vi "Helium Fridge Cool-Down.vi"() -> ()   [LabVIEW 2014]
uses:
  <vilib>/Analysis/8numeric.llb/1D Numeric Integration.vi
  <vilib>/express/express shared/transition.llb/Dynamic To Waveform Array.vi
  <vilib>/express/express signal manip/GetorSetDDTAttributes/Set DDT Attributes/SetT0.vi
  <vilib>/express/express shared/transition.llb/Waveform Array To Dynamic.vi
  <vilib>/express/express signal manip/GetorSetDDTAttributes/Set DDT Attributes/Set DDT Properties.xnode
  <vilib>/Analysis/NI_AALPro.lvlib
panel:
  out "Numeric Indicator":dbl
  in  "Depth/Div Submit":bool
  out "Depth/Div (kHz)":dbl
  in  "Cent. Frq. Submit":bool
  out "Cent. Freq. (MHz)":dbl
  out "Temp 2":bool
  out "Temperature Strip Chart":dynamicdata(graph)
  in  "TC Points/Measurement":dbl=20.0
  out "NMR":bool
  out "NMR Temp Error":bool
  out "Q Meter Temp":dynamicdata(graph)
  out "Zeroed Array":dbl[](array[numeric])
  out "Fit X values":dbl[](array[numeric])
  in  "Left wing 2":dbl
  in  "Right wing 2":dbl
  in  "Right wing":dbl
  in  "Left wing":dbl
  out "Fit":dbl[](array[numeric])
  in  "Submit":bool
  out "Is Flashing":bool
  in  "Error Beat":bool
  in  "Clear":bool
  in  "Comment":string
  out "Heartbeat":bool
  out "Most Recent Error":string
  out "Baseline Subtracted Integral vs. Time":dbl(graph)
  out "Time of Last Baseline":string
  out "Baseline":dbl[](array[numeric])
  in  "Baseline Subtract":bool
  in  "Get Baseline":bool
  out "Recording":bool
  out "Time of Last Recording":string
  in  "Record \nNMR Sweeps":bool
  in  "Depth/Div\n(MHz)":dbl=10.0
  in  "Central Freq. \n(MHz)":dbl=13.0
  in  "stop (F)":bool caption="Triangle Wave"
  in  "Triangle Wave\nRate (Hz)":dbl=0.3
  out "Time Elapsed \nDuring Sweeps (s)":dbl
  out "Lab Time":string
  out "Most Recent Error (NMR)":string
  out "Last Sweep Start Time":string
  out "Most Recent Error (Temp)":string
  out "Last Measurement Taken":string
  out "VI Start Time":string
  in  "Time Between\nTemp Ponts (s)":dbl=30.0
  out "Temp":bool
  out "NMR":bool
  in  "stop":bool
  out "Input Triangle Wave":dynamicdata(graph)
  out "Modulator":dynamicdata(graph)
  out "NMR":cluster{"Y":dbl[], "Y":dbl[]}[](graph)
  in  "# of Sweeps":dbl=1.0
  out "Resistance Strip Chart":dynamicdata(graph)
  in  "Heartbeat":bool
  in  "Temp Strip Chart":bool
  out "Errors":bool
  in  "Silence Flashing":bool
  # "Initialization and Logic Controls -- DO NOT TOUCH!!"
  # "Caitlyn's Work"
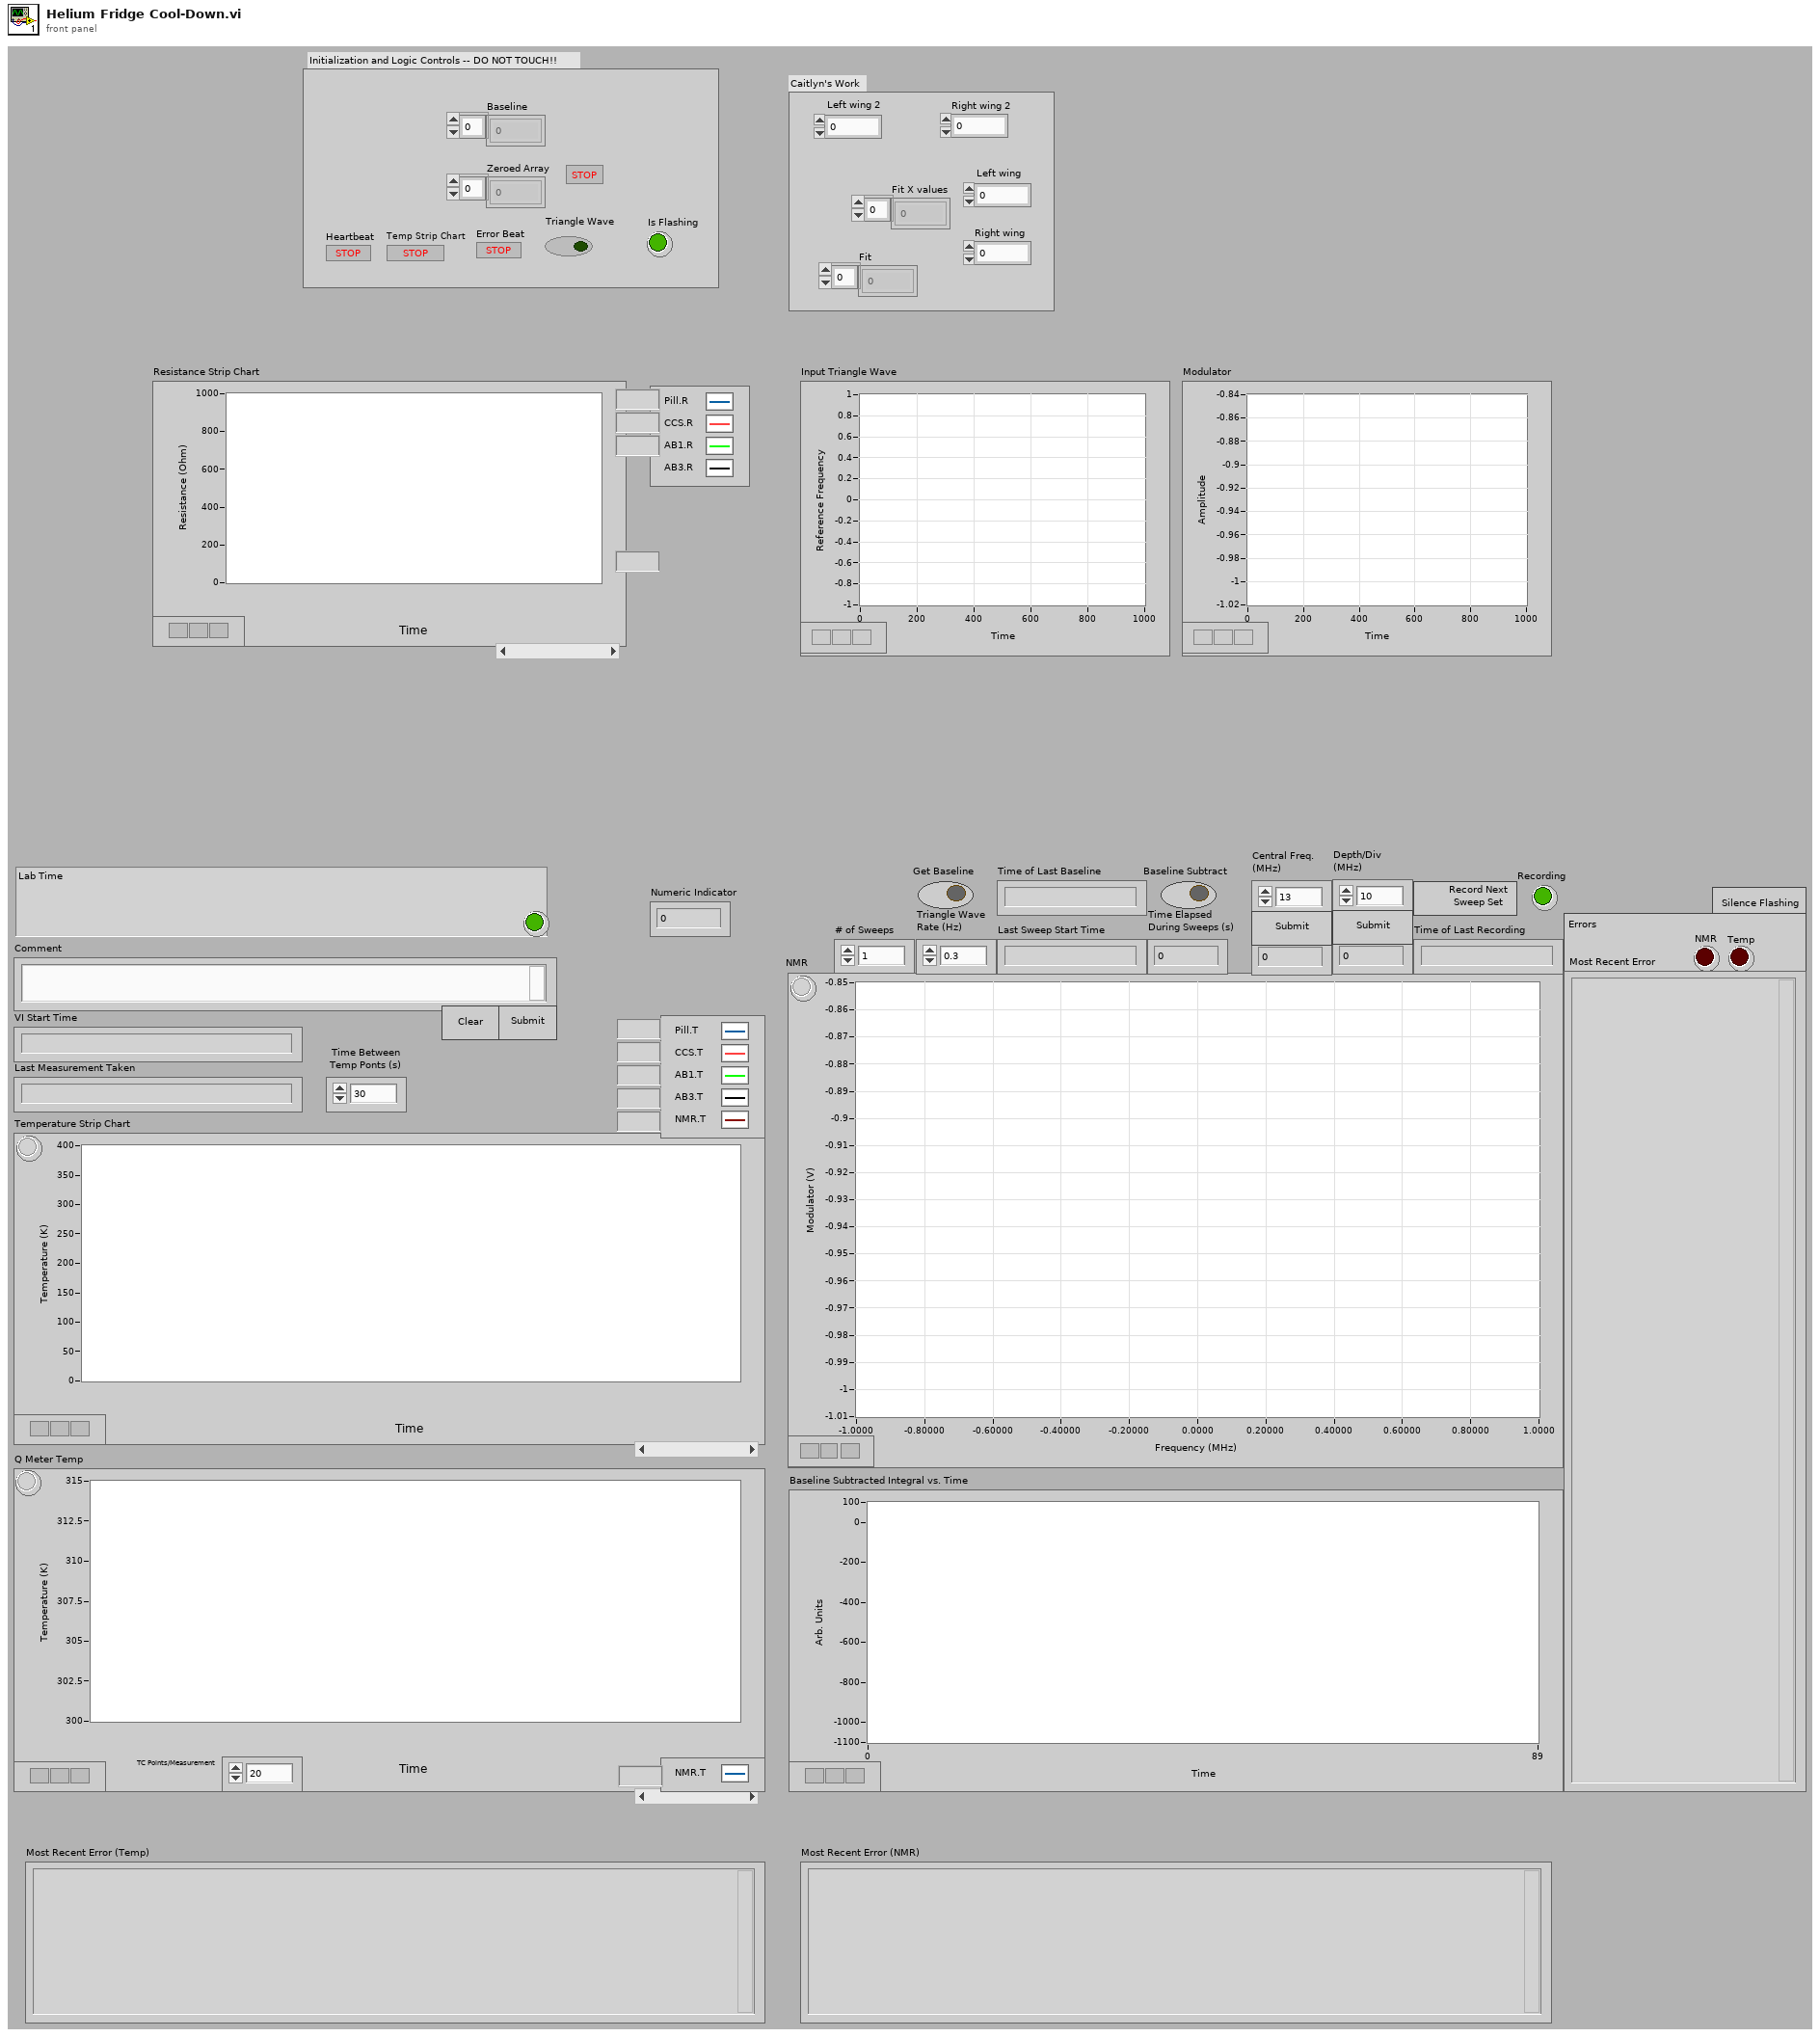
[diagram p1: front panel]
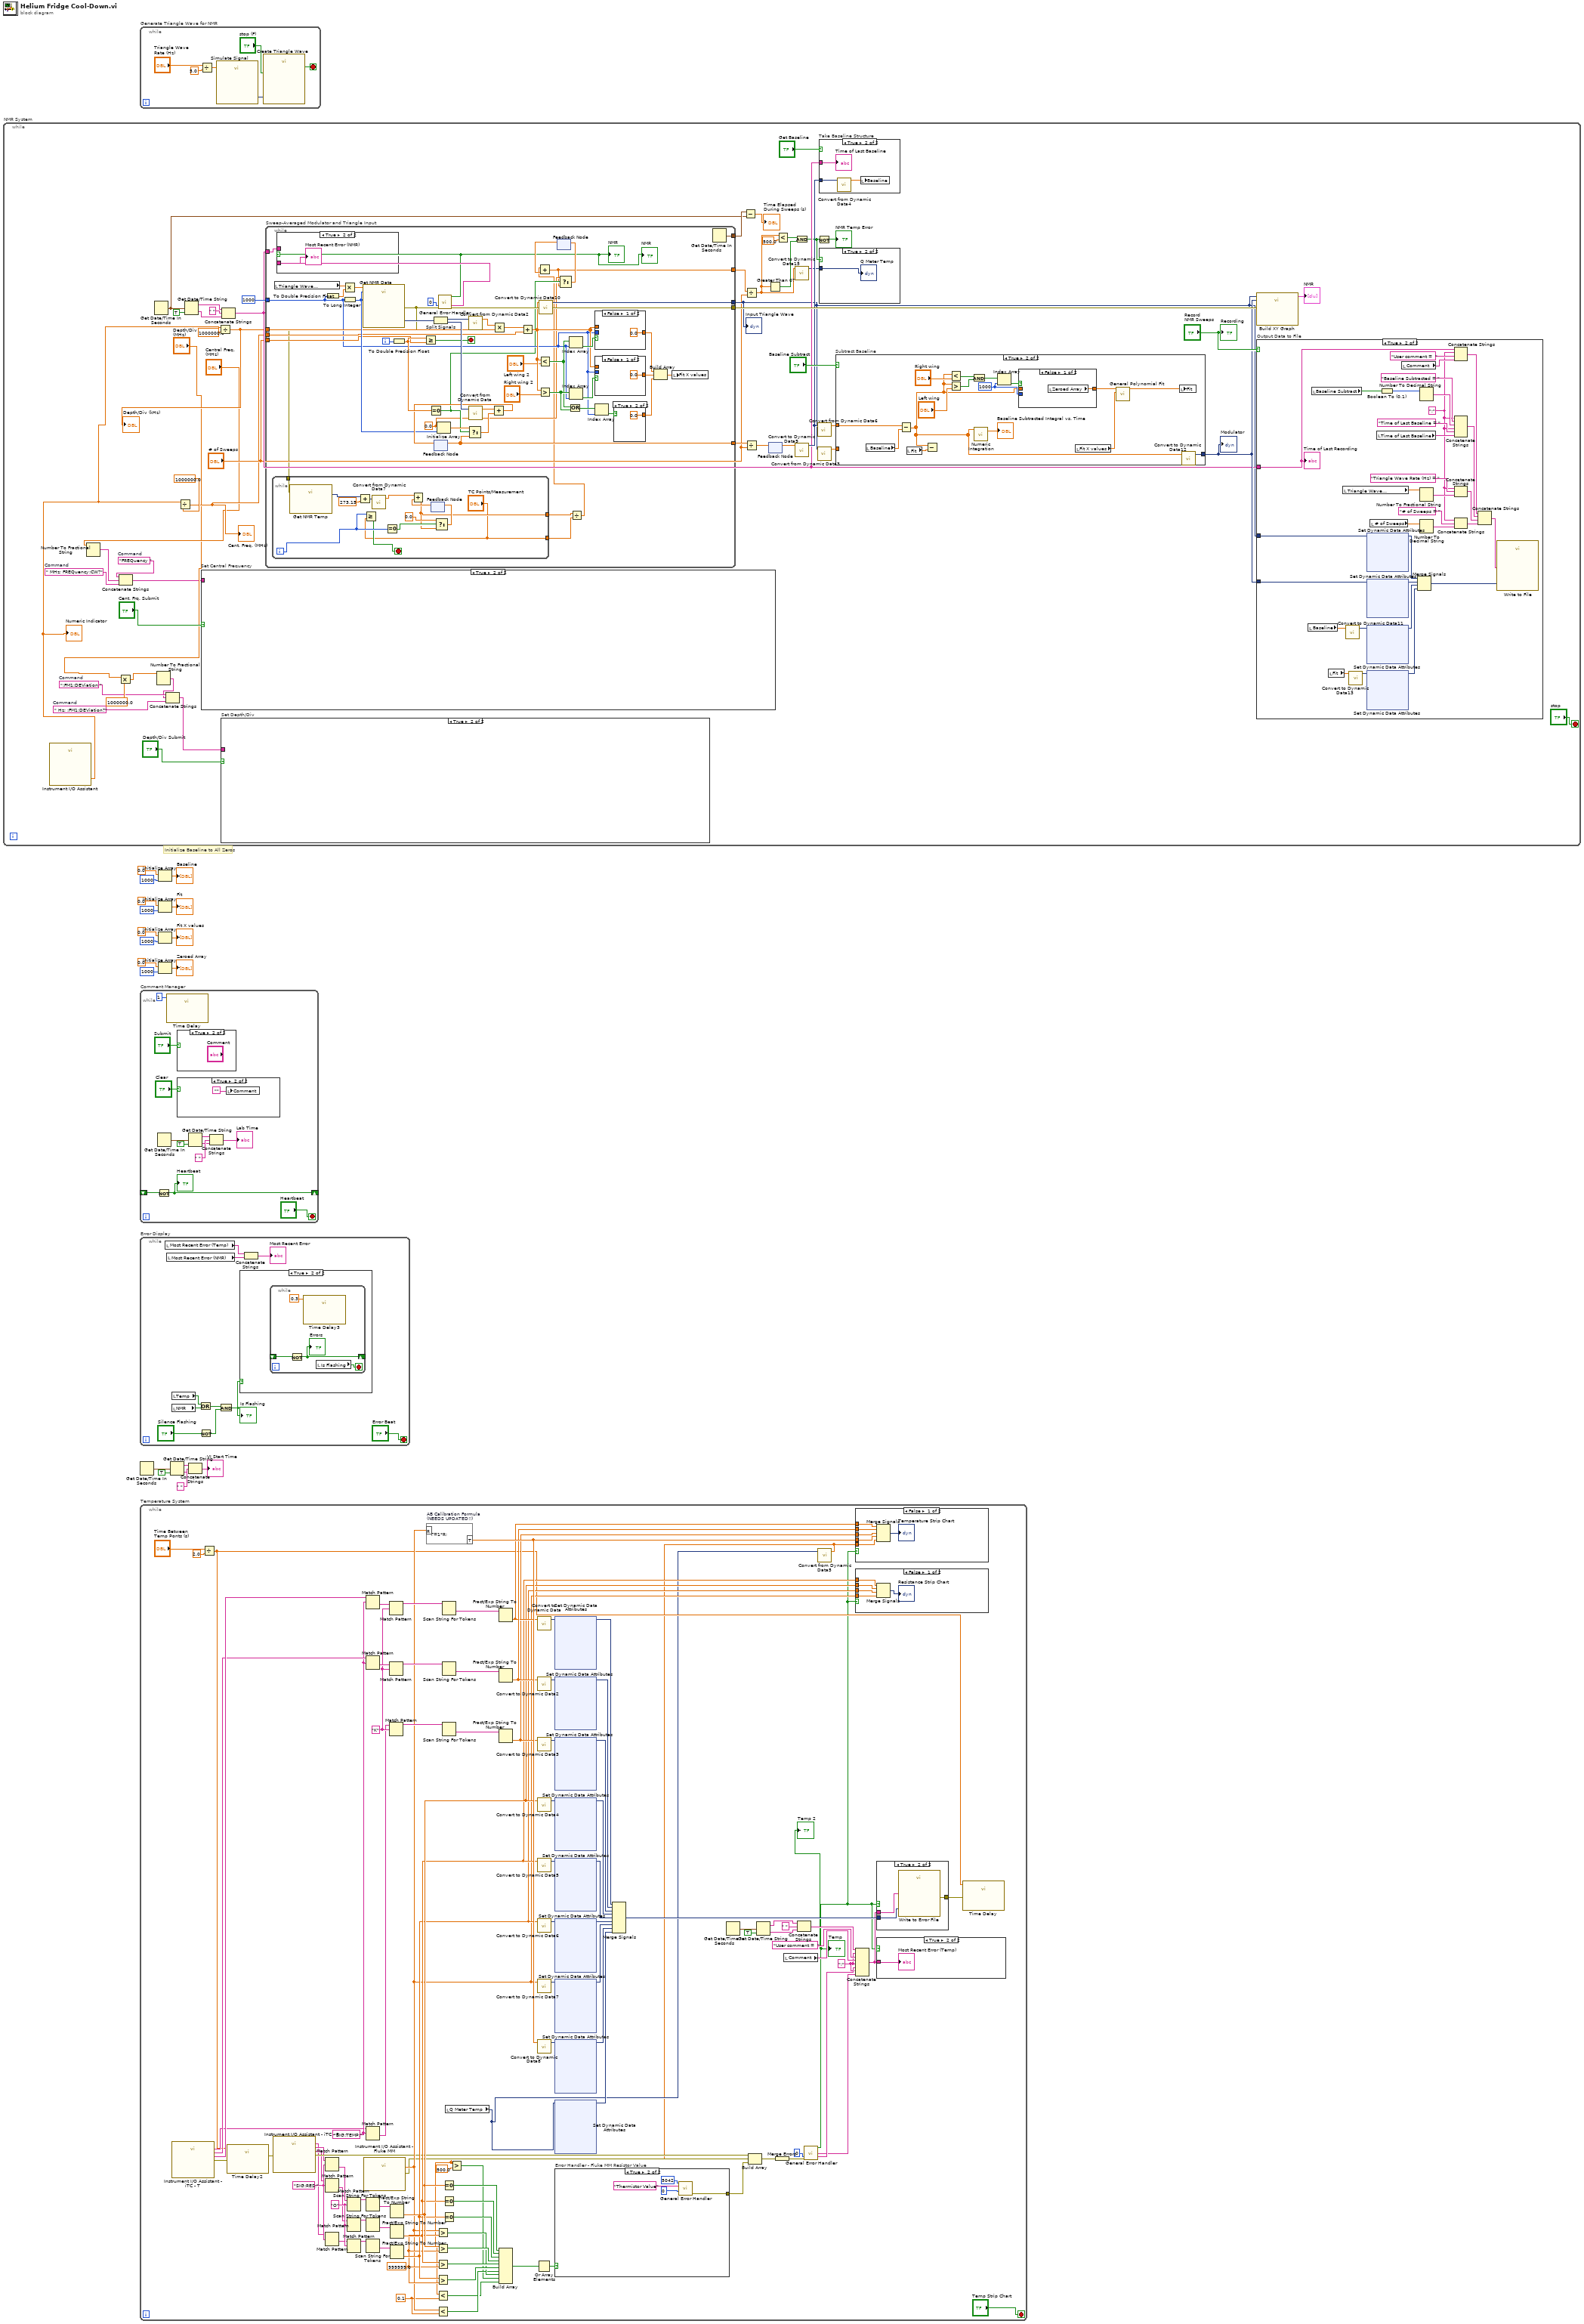
[diagram p0: block diagram]
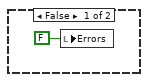
[diagram p2: hidden frame]
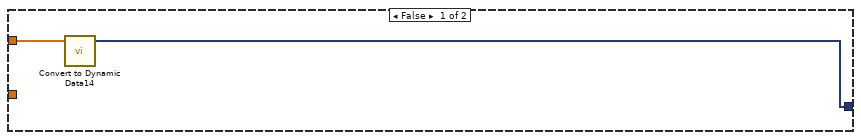
[diagram p6: hidden frame]
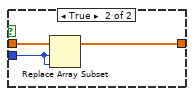
[diagram p7: hidden frame]
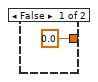
[diagram p10: hidden frame]
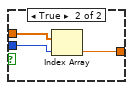
[diagram p11: hidden frame]
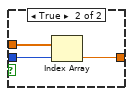
[diagram p12: hidden frame]
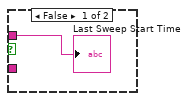
[diagram p13: hidden frame]
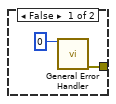
[diagram p16: hidden frame]
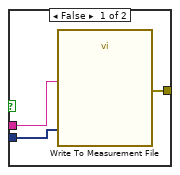
[diagram p19: hidden frame]
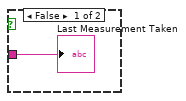
[diagram p20: hidden frame]
diagram:
  # "Initialize Baseline to All Zeros"
  n1 = while "NMR System" {
    stop <- "stop" stop-if-true
    w25 = " Hz; :FM1:DEViation?"  # Command
    w24 = ":FM1:DEViation "  # Command
    w30 = " MHz; FREQuency:CW?"  # Command
    w31 = "FREQuency "  # Command
    n2 = call "Instrument I/O Assistant"() -> ("CentralFreq"=w19:dbl)  [unwired: 25 in, 2 out]
    "Numeric Indicator" <- w19
    n3 = Number To Fractional String(number="Central Freq. \n(MHz)") -> (F-format string=w29:string)  [unwired: 3 in]
    n4 = Concatenate Strings(w31, w29, w30) -> (w21:string)
    n5 = Multiply(x="Depth/Div\n(MHz)", y=1000000.0) -> (x*y=w27:dbl)
    n6 = Get Date/Time In Seconds() -> (seconds since 1Jan1904=w58:timestamp)
    n7 = Number To Fractional String(number=w27) -> (F-format string=w20:string)  [unwired: 3 in]
    n8 = Concatenate Strings(w24, w20, w25) -> (w22:string)
    n9 = Divide(x=w19, y=1000000.0) -> (x/y=w34:dbl)
    "Cent. Freq. (MHz)" <- w34
    n10 = Get Date/Time String(seconds (now)=w58, want seconds? (F)=TRUE) -> (date string=w61:string, time string=w63:string)  [unwired: 1 in]
    n11 = case "Set Central Frequency" shown="True" "Cent. Frq. Submit" {
      tunnel: w21 -> [_ _]
      frame False {
      }
      frame True {
      }
    }
    n12 = Divide(x=w19, y=1000000.0) -> (x/y=w32:dbl)
    "Depth/Div (kHz)" <- w32
    n13 = case "Set Depth/Div" shown="True" "Depth/Div Submit" {
      tunnel: w22 -> [_ _]
      frame False {
      }
      frame True {
      }
    }
    n14 = Concatenate Strings(w61, " ", w63) -> (w49:string)
    n15 = while "Sweep-Averaged Modulator and Triangle Input" {
      tunnel: "# of Sweeps" -> [w224]
      tunnel: 1000 -> [w215]
      tunnel: [w241] -> w66
      tunnel: w49 -> [w237]
      tunnel: [w236] -> w59
      tunnel: [w234] -> w56
      tunnel: w32 -> [w228]
      tunnel: w34 -> [w226]
      tunnel: [w225] -> w48
      tunnel: [w205] -> w37
      i -> [w247]
      stop <- w240 stop-if-true
      w208 = 0.0
      n16 = local read "Triangle Wave\nRate (Hz)"() -> (w233:dbl)
      n17 = To Double Precision Float(number=w215) -> (double precision float=w231:dbl)
      n18 = Multiply(x=w233, y=w231) -> (x*y=w235:dbl)
      n19 = To Long Integer(number=w215) -> (32bit integer=w232:i32)
      n20 = call "Get NMR Data"("rate"=w235, "number of samples"=w232) -> ("data"=w249:dynamicdata, "error out"=w200:errorcluster)  [unwired: 15 in, 1 out]
      n21 = while {
        tunnel: ["TC Points/Measurement"] -> w203
        tunnel: [w254] -> w202
        tunnel: w200 -> [w253]
        i -> [w252]
        stop <- w251 stop-if-true
        n22 = call "Get NMR Temp"("error in"=w253) -> ("data"=w256:dynamicdata)  [unwired: 16 in, 2 out]
        n23 = Add(x=w256, y=273.15) -> (x+y=w255:dynamicdata)
        n24 = Greater Or Equal?(x=w252, y="TC Points/Measurement") -> (x >= y?=w251:bool)
        n25 = call "Convert from Dynamic Data7"("Dynamic Data Type"=w255) -> ("Scalar"=w258:dbl)  [unwired: 3 in]
        n26 = Equal To 0?(x=w252) -> (x = 0?=w259:bool)
        n27 = feedback #1() -> (w261:dbl)  [unwired: 1 in]
        n28 = Add(x=w258, y=w261) -> (x+y=w254:dbl)
        n29 = Select(t=0.0, s=w259, f=w254) -> (s? t:f=w260:dbl)
        n30 = feedback-in #1(w260) -> ()
      }
      n31 = To Double Precision Float(number=w247) -> (double precision float=w246:dbl)
      n32 = Greater Or Equal?(x=w246, y=w224) -> (x >= y?=w240:bool)
      n33 = Equal To 0?(x=w246) -> (x = 0?=w209:bool)
      n34 = Split Signals(w249) -> (w230:dynamicdata, w248:dynamicdata)  [unwired: 2 in]
      n35 = feedback #2() -> (w241:dbl[])  [unwired: 1 in]
      n36 = Initialize Array(w208, w232) -> (w244:dbl[])
      n37 = call <vilib>:"General Error Handler.vi"("type of dialog (OK msg:1)"=0, "error in (no error)"=w200) -> ("error?"=w204:bool, "message"=w239:string, "error out"=w234:errorcluster)  [unwired: 9 in, 2 out]
      "NMR" <- w204
      "NMR" <- w204
      n38 = case shown="True" w204 {
        tunnel: w239 -> [_ w274]
        tunnel: w237 -> [w273 _]
        frame False {
          "Last Sweep Start Time" <- w273
        }
        frame True {
          "Most Recent Error (NMR)" <- w274
        }
      }
      n39 = call "Convert from Dynamic Data2"("Dynamic Data Type"=w230) -> ("Array"=w229:dbl[])  [unwired: 3 in]
      n40 = call "Convert from Dynamic Data"("Dynamic Data Type"=w248) -> ("Array"=w243:dbl[])  [unwired: 3 in]
      n41 = Select(t=w244, s=w209, f=w241) -> (s? t:f=w245:dbl[])
      n42 = Add(x=w243, y=w245) -> (x+y=w242:dbl[])
      n43 = feedback-in #2(w242) -> ()
      n44 = Multiply(x=w229, y=w228) -> (x*y=w227:dbl[])
      n45 = Add(x=w227, y=w226) -> (x+y=w221:dbl[])
      n46 = Less?(x=w221, y="Left wing 2") -> (x < y?=w217:bool[])
      n47 = Greater?(x=w221, y="Right wing 2") -> (0:w218:bool[])
      n48 = call "Convert to Dynamic Data10"("Array"=w221) -> ("Dynamic Data Type"=w225:dynamicdata)  [unwired: 3 in]
      n49 = feedback #3() -> (w206:dbl)  [unwired: 1 in]
      n50 = Or(x=w217, y=w218) -> (x .or. y?=w216:bool[])
      n51 = Index Array(array=w217, index=w215) -> (element=w223:bool)
      n52 = Index Array(array=w218, index=w215) -> (element=w222:bool)
      n53 = Divide(x=w202, y=w203) -> (x/y=w201:dbl)
      n54 = Add(x=w201, y=w206) -> (x+y=w205:dbl)
      n55 = Select(t=w208, s=w209, f=w205) -> (s? t:f=w207:dbl)
      n56 = feedback-in #3(w207) -> ()
      n57 = case shown="False" w223 {
        tunnel: w221 -> [_ w272]
        tunnel: w215 -> [_ w271]
        tunnel: [0.0 w270] -> w219
        frame False {
        }
        frame True {
          n58 = Index Array(array=w272, index=w271) -> (element=w270:dbl)
        }
      }
      n59 = case shown="False" w222 {
        tunnel: w221 -> [_ w268]
        tunnel: w215 -> [_ w267]
        tunnel: [0.0 w266] -> w220
        frame False {
        }
        frame True {
          n60 = Index Array(array=w268, index=w267) -> (element=w266:dbl)
        }
      }
      n61 = Index Array(array=w216, index=w215) -> (element=w214:bool)
      n62 = case shown="True" w214 {
        tunnel: [0.0 0.0] -> w213
        frame False {
        }
        frame True {
        }
      }
      n63 = Build Array(w219, w220, w213) -> (w210:dbl[])
      n64 = local write "Fit X values"(w210) -> ()
      n65 = Get Date/Time In Seconds() -> (seconds since 1Jan1904=w236:timestamp)
    }
    "Input Triangle Wave" <- w48
    n66 = Subtract(x=w59, y=w58) -> (x-y=→"Time Elapsed \nDuring Sweeps (s)":dbl)
    n67 = Divide(x=w37, y="# of Sweeps") -> (x/y=w38:dbl)
    n68 = Divide(x=w66, y="# of Sweeps") -> (x/y=w65:dbl[])
    n69 = Greater Than 0?(x=w38) -> (x > 0?=w45:bool)
    n70 = feedback-in #4(w65) -> ()
    n71 = feedback #4() -> (w64:dbl[])  [unwired: 1 in]
    n72 = Less?(x=w38, y=500.0) -> (x < y?=w42:bool)
    n73 = And(x=w42, y=w45) -> (x .and. y?=w44:bool)
    n74 = call "Convert to Dynamic Data15"("Double"=w38) -> ("Dynamic Data Type"=w40:dynamicdata)  [unwired: 3 in]
    n75 = call "Convert to Dynamic Data9"("Array"=w64) -> ("Dynamic Data Type"=w51:dynamicdata)  [unwired: 3 in]
    n76 = Not(x=w44) -> (.not. x?=→"NMR Temp Error":bool)
    n77 = call "Convert from Dynamic Data6"("Dynamic Data Type"=w51) -> ("Array"=w46:dbl[])  [unwired: 3 in]
    n78 = call "Convert from Dynamic Data3"("Dynamic Data Type"=w48) -> ("Array"=w47:dbl[])  [unwired: 3 in]
    n79 = case "Take Baseline Structure" shown="True" "Get Baseline" {
      tunnel: w51 -> [_ w95]
      tunnel: w49 -> [_ w93]
      frame False {
      }
      frame True {
        n80 = call "Convert from Dynamic Data4"("Dynamic Data Type"=w95) -> ("Array"=w94:dbl[])  [unwired: 3 in]
        n81 = local write "Baseline"(w94) -> ()
        "Time of Last Baseline" <- w93
      }
    }
    n82 = case shown="True" w44 {
      tunnel: w40 -> [_ w70]
      frame False {
      }
      frame True {
        "Q Meter Temp" <- w70
      }
    }
    n83 = case "Subtract Baseline" shown="True" "Baseline Subtract" {
      tunnel: w46 -> [w72 w88]
      tunnel: [w71 w87] -> w50
      tunnel: w47 -> [_ _]
      frame False {
        n84 = call "Convert to Dynamic Data14"("Array"=w72) -> ("Dynamic Data Type"=w71:dynamicdata)  [unwired: 3 in]
      }
      frame True {
        w77 = 1000
        n85 = local read "Baseline"() -> (w85:dbl[])
        n86 = Subtract(x=w88, y=w85) -> (x-y=w73:dbl[])
        n87 = local read "Fit"() -> (w84:dbl[])
        n88 = Subtract(x=w73, y=w84) -> ()  [unwired: 1 out]
        n89 = Less?(x=w73, y="Right wing") -> (x < y?=w81:bool[])
        n90 = Greater?(x=w73, y="Left wing") -> (0:w80:bool[])
        n91 = And(x=w81, y=w80) -> (x .and. y?=w79:bool[])
        n92 = call-poly <vilib>:"Numeric Integration.vi"("Input Array"=w73) -> ("result"=→"Baseline Subtracted Integral vs. Time":dbl)  [unwired: 2 in, 1 out]
        n93 = Index Array(array=w79, index=w77) -> (element=w78:bool)
        n94 = case shown="False" w78 {
          tunnel: w73 -> [_ w92]
          tunnel: w77 -> [_ w90]
          tunnel: [w89 w91] -> w76
          frame False {
            n95 = local read "Zeroed Array"() -> (w89:dbl[])
          }
          frame True {
            n96 = Replace Array Subset(array=w92, new element=w90, index=w90) -> (w91:dbl[])
          }
        }
        n97 = local read "Fit X values"() -> (w74:dbl[])
        n98 = call <vilib>:"General Polynomial Fit.vi"("Y"=w76, "X"=w74) -> ("Best Polynomial Fit"=w75:dbl[])  [unwired: 10 in, 3 out]
        n99 = local write "Fit"(w75) -> ()
        n100 = call "Convert to Dynamic Data12"("Array"=w73) -> ("Dynamic Data Type"=w87:dynamicdata)  [unwired: 3 in]
      }
    }
    "Modulator" <- w50
    n101 = call "Build XY Graph"("error in (no error)"=w56, "Y Input"=w50, "X Input"=w48) -> ("XY Graph"=→"NMR":cluster{"Y":dbl[], "Y":dbl[]}[])  [unwired: 7 in, 1 out]
    n102 = case "Output Data to File" shown="True" "Record \nNMR Sweeps" {
      tunnel: w49 -> [_ w116]
      tunnel: w50 -> [_ w123]
      tunnel: w48 -> [_ w122]
      frame False {
      }
      frame True {
        w100 = ";"
        n103 = local read "Baseline"() -> (w121:dbl[])
        n104 = local read "Baseline Subtract"() -> (w118:bool)
        n105 = local read "Fit"() -> (w99:dbl[])
        n106 = local read "Triangle Wave\nRate (Hz)"() -> (w119:dbl)
        n107 = call "Convert to Dynamic Data11"("Array"=w121) -> ("Dynamic Data Type"=w120:dynamicdata)  [unwired: 3 in]
        n108 = call "Convert to Dynamic Data13"("Array"=w99) -> ("Dynamic Data Type"=w98:dynamicdata)  [unwired: 3 in]
        n109 = xnode "Set Dynamic Data Attributes"("Signals In"=w122) -> ("Signals Out"=w127:dynamicdata)  [unwired: 4 in, 1 out]
        n110 = xnode "Set Dynamic Data Attributes"("Signals In"=w123) -> ("Signals Out"=w125:dynamicdata)  [unwired: 4 in, 1 out]
        n111 = xnode "Set Dynamic Data Attributes"("Signals In"=w120) -> ("Signals Out"=w97:dynamicdata)  [unwired: 4 in, 1 out]
        n112 = xnode "Set Dynamic Data Attributes"("Signals In"=w98) -> ("Signals Out"=w96:dynamicdata)  [unwired: 4 in, 1 out]
        n113 = local read "# of Sweeps"() -> (w124:dbl)
        n114 = local read "Time of Last Baseline"() -> (w105:string)
        n115 = Boolean To (0,1)(Boolean=w118) -> (0, 1=w117:i16)
        n116 = local read "Comment"() -> (w114:string)
        n117 = Merge Signals(w127, w125, w97, w96) -> (w126:dynamicdata)
        n118 = Number To Decimal String(number=w117) -> (decimal integer string=w110:string)  [unwired: 1 in]
        n119 = Number To Fractional String(number=w119) -> (F-format string=w108:string)  [unwired: 3 in]
        n120 = Number To Decimal String(number=w124) -> (decimal integer string=w112:string)  [unwired: 1 in]
        n121 = Concatenate Strings(w116, w100, "User comment =  ", w114) -> (w107:string)
        n122 = Concatenate Strings(w100, "Baseline Subtracted = ", w110, w100, "Time of Last Baseline = ", w105) -> (w104:string)
        n123 = Concatenate Strings(w100, "Triangle Wave Rate (Hz) = ", w108) -> (w103:string)
        n124 = Concatenate Strings(w100, "# of Sweeps = ", w112) -> (w102:string)
        n125 = Concatenate Strings(w107, w104, w103, w102) -> (w101:string)
        n126 = call "Write to File"("Signals"=w126, "Comment"=w101) -> ()  [unwired: 15 in, 3 out]
        "Time of Last Recording" <- w116
      }
    }
    "Recording" <- "Record \nNMR Sweeps"
  }
  n127 = while "Generate Triangle Wave for NMR" {
    stop <- w279 stop-if-true
    n128 = Divide(x="Triangle Wave\nRate (Hz)", y=5.0) -> (x/y=w275:dbl)
    n129 = call "Simulate Signal"("Frequency"=w275) -> ("Triangle"=w278:dynamicdata)  [unwired: 13 in, 1 out]
    n130 = call "Create Triangle Wave"("data"=w278, "stop (F)"="stop (F)") -> ("stopped"=w279:bool)  [unwired: 15 in, 2 out]
  }
  n131 = while "Comment Manager" {
    shift-right: [w289] -> _
    shift-left: _ -> [w292]
    stop <- "Heartbeat" stop-if-true
    n132 = Not(x=w292) -> (.not. x?=w289:bool)
    "Heartbeat" <- w289
    n133 = Get Date/Time In Seconds() -> (seconds since 1Jan1904=w287:timestamp)
    n134 = call "Time Delay"("Delay Time (s)"=1) -> ()  [unwired: 10 in, 1 out]
    n135 = case shown="True" "Submit" {
      frame False {
      }
      frame True {
      }
    }
    n136 = case shown="True" "Clear" {
      frame False {
      }
      frame True {
        n137 = local write "Comment"("") -> ()
      }
    }
    n138 = Get Date/Time String(seconds (now)=w287, want seconds? (F)=TRUE) -> (date string=w286:string, time string=w284:string)  [unwired: 1 in]
    n139 = Concatenate Strings(w286, " ", w284) -> (→"Lab Time":string)
  }
  n140 = while "Error Display" {
    stop <- "Error Beat" stop-if-true
    n141 = local read "Most Recent Error (Temp)"() -> (w294:string)
    n142 = local read "Most Recent Error (NMR)"() -> (w295:string)
    n143 = local read "Temp"() -> (w303:bool)
    n144 = local read "NMR"() -> (w302:bool)
    n145 = Or(x=w303, y=w302) -> (x .or. y?=w300:bool)
    n146 = Not(x="Silence Flashing") -> (.not. x?=w298:bool)
    n147 = And(x=w300, y=w298) -> (x .and. y?=w297:bool)
    "Is Flashing" <- w297
    n148 = case shown="True" w297 {
      frame False {
        n149 = local write "Errors"(FALSE) -> ()
      }
      frame True {
        n150 = while {
          shift-right: [w306] -> _
          shift-left: _ -> [w308]
          stop <- w305 stop-if-true
          n151 = Not(x=w308) -> (.not. x?=w306:bool)
          "Errors" <- w306
          n152 = call "Time Delay3"("Delay Time (s)"=0.3) -> ()  [unwired: 10 in, 1 out]
          n153 = local read "Is Flashing"() -> (w305:bool)
        }
      }
    }
    n154 = Concatenate Strings(w294, w295) -> (→"Most Recent Error":string)
  }
  n155 = Get Date/Time In Seconds() -> (seconds since 1Jan1904=w17:timestamp)
  n156 = while "Temperature System" {
    stop <- "Temp Strip Chart" stop-if-true
    w317 = ";"
    w313 = 0.1
    w339 = 999999.0
    w375 = "O"
    w376 = "SIG:RES:"
    w382 = "SIG:TEMP:"
    w381 = "K"
    n157 = call "Instrument I/O Assistant - iTC - T"() -> ("AB1.T"=w380:string, "CCS.T"=w385:string, "Pill.T"=w388:string, "error out"=w330:errorcluster)  [unwired: 23 in, 1 out]
    n158 = Divide(x="Time Between\nTemp Ponts (s)", y=2.0) -> (x/y=w325:dbl)
    n159 = call "Time Delay2"("error in (no error)"=w330, "Delay Time (s)"=w325) -> ("error out"=w331:errorcluster)  [unwired: 9 in]
    n160 = call "Instrument I/O Assistant - iTC - R"("error in"=w331) -> ("AB1.R"=w327:string, "CCS.R"=w328:string, "Pill.R"=w329:string, "error out"=w332:errorcluster)  [unwired: 22 in, 1 out]
    n161 = Match Pattern(string=w328, regular expression=w376) -> (after substring=w374:string)  [unwired: 1 in, 3 out]
    n162 = Match Pattern(string=w329, regular expression=w376) -> (after substring=w373:string)  [unwired: 1 in, 3 out]
    n163 = Match Pattern(string=w327, regular expression=w376) -> (after substring=w372:string)  [unwired: 1 in, 3 out]
    n164 = Match Pattern(string=w374, regular expression=w375) -> (before substring=w371:string)  [unwired: 1 in, 3 out]
    n165 = Match Pattern(string=w373, regular expression=w375) -> (before substring=w370:string)  [unwired: 1 in, 3 out]
    n166 = Match Pattern(string=w372, regular expression=w375) -> (before substring=w369:string)  [unwired: 1 in, 3 out]
    n167 = call "Instrument I/O Assistant - Fluke MM"() -> ("AB3.R"=w337:dbl, "error out"=w335:errorcluster)  [unwired: 25 in, 1 out]
    n168 = Match Pattern(string=w388, regular expression=w382) -> (after substring=w387:string)  [unwired: 1 in, 3 out]
    n169 = Match Pattern(string=w385, regular expression=w382) -> (after substring=w384:string)  [unwired: 1 in, 3 out]
    n170 = Match Pattern(string=w380, regular expression=w382) -> (after substring=w379:string)  [unwired: 1 in, 3 out]
    n171 = Scan String For Tokens(9:w371) -> (1:w368:string)  [unwired: 5 in, 3 out]
    n172 = Scan String For Tokens(9:w370) -> (1:w367:string)  [unwired: 5 in, 3 out]
    n173 = Scan String For Tokens(9:w369) -> (1:w366:string)  [unwired: 5 in, 3 out]
    n174 = Match Pattern(string=w387, regular expression=w381) -> (before substring=w386:string)  [unwired: 1 in, 3 out]
    n175 = Match Pattern(string=w384, regular expression=w381) -> (before substring=w383:string)  [unwired: 1 in, 3 out]
    n176 = Match Pattern(string=w379, regular expression=w381) -> (before substring=w378:string)  [unwired: 1 in, 3 out]
    n177 = Fract/Exp String To Number(string=w368) -> (number=w345:dbl)  [unwired: 3 in, 1 out]
    n178 = Fract/Exp String To Number(string=w367) -> (number=w344:dbl)  [unwired: 3 in, 1 out]
    n179 = Fract/Exp String To Number(string=w366) -> (number=w343:dbl)  [unwired: 3 in, 1 out]
    n180 = formula code="T=1*R;" "AB Calibration Formula\n(NEEDS UPDATED!!)"("R"=w337) -> ("T"=w356:dbl)
    n181 = Greater?(x=w337, y=w339) -> (0:w338:bool)
    n182 = Greater?(x=w345, y=w339) -> (0:w342:bool)
    n183 = Greater?(x=w344, y=w339) -> (0:w341:bool)
    n184 = Greater?(x=w343, y=w339) -> (0:w340:bool)
    n185 = Less?(x=w337, y=w313) -> (x < y?=w336:bool)
    n186 = Scan String For Tokens(9:w386) -> (1:w405:string)  [unwired: 5 in, 3 out]
    n187 = Scan String For Tokens(9:w383) -> (1:w403:string)  [unwired: 5 in, 3 out]
    n188 = Scan String For Tokens(9:w378) -> (1:w402:string)  [unwired: 5 in, 3 out]
    n189 = Equal To 0?(x=w345) -> (x = 0?=w353:bool)
    n190 = Equal To 0?(x=w344) -> (x = 0?=w352:bool)
    n191 = Equal To 0?(x=w343) -> (x = 0?=w351:bool)
    n192 = local read "Q Meter Temp"() -> (w310:dynamicdata)
    n193 = Fract/Exp String To Number(string=w405) -> (number=w347:dbl)  [unwired: 3 in, 1 out]
    n194 = Fract/Exp String To Number(string=w403) -> (number=w348:dbl)  [unwired: 3 in, 1 out]
    n195 = Fract/Exp String To Number(string=w402) -> (number=w346:dbl)  [unwired: 3 in, 1 out]
    n196 = call "Convert to Dynamic Data"("Double"=w347) -> ("Dynamic Data Type"=w396:dynamicdata)  [unwired: 3 in]
    n197 = call "Convert to Dynamic Data2"("Double"=w348) -> ("Dynamic Data Type"=w394:dynamicdata)  [unwired: 3 in]
    n198 = call "Convert to Dynamic Data3"("Double"=w346) -> ("Dynamic Data Type"=w393:dynamicdata)  [unwired: 3 in]
    n199 = call "Convert to Dynamic Data4"("Double"=w345) -> ("Dynamic Data Type"=w365:dynamicdata)  [unwired: 3 in]
    n200 = call "Convert to Dynamic Data5"("Double"=w344) -> ("Dynamic Data Type"=w364:dynamicdata)  [unwired: 3 in]
    n201 = call "Convert to Dynamic Data6"("Double"=w343) -> ("Dynamic Data Type"=w363:dynamicdata)  [unwired: 3 in]
    n202 = call "Convert to Dynamic Data7"("Double"=w337) -> ("Dynamic Data Type"=w359:dynamicdata)  [unwired: 3 in]
    n203 = call "Convert to Dynamic Data8"("Double"=w356) -> ("Dynamic Data Type"=w355:dynamicdata)  [unwired: 3 in]
    n204 = xnode "Set Dynamic Data Attributes"("Signals In"=w396) -> ("Signals Out"=w395:dynamicdata)  [unwired: 4 in, 1 out]
    n205 = xnode "Set Dynamic Data Attributes"("Signals In"=w394) -> ("Signals Out"=w392:dynamicdata)  [unwired: 4 in, 1 out]
    n206 = xnode "Set Dynamic Data Attributes"("Signals In"=w393) -> ("Signals Out"=w391:dynamicdata)  [unwired: 4 in, 1 out]
    n207 = xnode "Set Dynamic Data Attributes"("Signals In"=w365) -> ("Signals Out"=w362:dynamicdata)  [unwired: 4 in, 1 out]
    n208 = xnode "Set Dynamic Data Attributes"("Signals In"=w364) -> ("Signals Out"=w361:dynamicdata)  [unwired: 4 in, 1 out]
    n209 = xnode "Set Dynamic Data Attributes"("Signals In"=w363) -> ("Signals Out"=w360:dynamicdata)  [unwired: 4 in, 1 out]
    n210 = xnode "Set Dynamic Data Attributes"("Signals In"=w359) -> ("Signals Out"=w358:dynamicdata)  [unwired: 4 in, 1 out]
    n211 = xnode "Set Dynamic Data Attributes"("Signals In"=w355) -> ("Signals Out"=w354:dynamicdata)  [unwired: 4 in, 1 out]
    n212 = xnode "Set Dynamic Data Attributes"("Signals In"=w310) -> ("Signals Out"=w316:dynamicdata)  [unwired: 4 in, 1 out]
    n213 = Merge Signals(w395, w392, w391, w362, w361, w360, w358, w354, w316) -> (w390:dynamicdata)
    n214 = Get Date/Time In Seconds() -> (seconds since 1Jan1904=w401:timestamp)
    n215 = Get Date/Time String(seconds (now)=w401, want seconds? (F)=TRUE) -> (date string=w399:string, time string=w397:string)  [unwired: 1 in]
    n216 = local read "Comment"() -> (w322:string)
    n217 = Concatenate Strings(w399, " ", w397) -> (w318:string)
    n218 = call "Convert from Dynamic Data5"("Dynamic Data Type"=w310) -> ("Scalar"=w309:dbl)  [unwired: 3 in]
    n219 = Less?(x=w309, y=w313) -> (x < y?=w312:bool)
    n220 = Greater?(x=w309, y=500.0) -> (0:w314:bool)
    n221 = Build Array(w353, w352, w351, w342, w341, w340, w336, w338, w314, w312) -> (w350:bool[])
    n222 = Or Array Elements(Boolean array=w350) -> (logical OR=w349:bool)
    n223 = case "Error Handler - Fluke MM Resistor Value" shown="True" w349 {
      tunnel: [w424 w429] -> w334
      frame False {
        n224 = call <vilib>:"General Error Handler.vi"("[error code] (0)"=0) -> ("error out"=w424:errorcluster)  [unwired: 10 in, 4 out]
      }
      frame True {
        n225 = call <vilib>:"General Error Handler.vi"("[error code] (0)"=5042, "[error source] (\" \")"="Thermistor Value", "type of dialog (OK msg:1)"=0) -> ("error out"=w429:errorcluster)  [unwired: 8 in, 4 out]
      }
    }
    n226 = Build Array(w332, w335, w334) -> (w333:errorcluster[])
    n227 = Merge Errors(w333) -> (w357:errorcluster)
    n228 = call <vilib>:"General Error Handler.vi"("type of dialog (OK msg:1)"=0, "error in (no error)"=w357) -> ("error?"=w311:bool, "source out"=w319:string, "message"=w321:string)  [unwired: 9 in, 2 out]
    "Temp" <- w311
    "Temp 2" <- w311
    n229 = case shown="False" w311 {
      tunnel: w347 -> [w530 _]
      tunnel: w348 -> [w529 _]
      tunnel: w346 -> [w528 _]
      tunnel: w356 -> [w527 _]
      tunnel: w309 -> [w525 _]
      frame False {
        n230 = Merge Signals(w530, w529, w528, w527, w525) -> (→"Temperature Strip Chart":dynamicdata)
      }
      frame True {
      }
    }
    n231 = case shown="False" w311 {
      tunnel: w344 -> [w524 _]
      tunnel: w345 -> [w523 _]
      tunnel: w343 -> [w522 _]
      tunnel: w337 -> [w521 _]
      frame False {
        n232 = Merge Signals(w524, w523, w522, w521) -> (→"Resistance Strip Chart":dynamicdata)
      }
      frame True {
      }
    }
    n233 = Concatenate Strings(w318, w317, "User comment =  ", w322, w317, w321, w317, w319) -> (w320:string)
    n234 = case shown="True" w311 {
      tunnel: w390 -> [w533 w536]
      tunnel: w320 -> [w532 w535]
      tunnel: [w531 w534] -> w377
      frame False {
        n235 = call "Write To Measurement File"("Signals"=w533, "Comment"=w532) -> ("error out"=w531:errorcluster)  [unwired: 15 in, 2 out]
      }
      frame True {
        n236 = call "Write to Error File"("Signals"=w536, "Comment"=w535) -> ("error out"=w534:errorcluster)  [unwired: 15 in, 2 out]
      }
    }
    n237 = case shown="True" w311 {
      tunnel: w320 -> [w591 w592]
      frame False {
        "Last Measurement Taken" <- w591
      }
      frame True {
        "Most Recent Error (Temp)" <- w592
      }
    }
    n238 = call "Time Delay"("error in (no error)"=w377, "Delay Time (s)"=w325) -> ()  [unwired: 9 in, 1 out]
  }
  n239 = Initialize Array(0.0, 1000) -> (→"Baseline":dbl[])
  n240 = Initialize Array(0.0 ("number"), 1000) -> (→"Fit":dbl[])
  n241 = Initialize Array(0.0, 1000) -> (→"Fit X values":dbl[])
  n242 = Initialize Array(0.0, 1000) -> (→"Zeroed Array":dbl[])
  n243 = Get Date/Time String(seconds (now)=w17, want seconds? (F)=TRUE) -> (date string=w16:string, time string=w14:string)  [unwired: 1 in]
  n244 = Concatenate Strings(w16, " ", w14) -> (→"VI Start Time":string)
